vi "Read.vi"(5 "CS Channel":u8, 7 "SPI Channel (0)":u8, 8 "Error In":errorcluster, 10 "LEDs":enum16{"None", "LD1", "LD2", "Both"}(ring)=enum."LD2", 11 "LINX Resource":T1) -> (0 "Error Out":errorcluster, 1 "Y - Axis":string, 2 "X - Axis":string, 3 "LINX Resource":T1, 4 "Buttons":u8)   [LabVIEW 2020, in "LMH-LINX.lvlib" / "PmodJSTK.lvlib"]
doc: "Sets the state of the LEDs on the PmodJSTK and reads X and Y axis data and button values."
uses:
  PmodJSTK.lvlib
  Private/Type Defs/LINX Ref.ctl
  Private/Type Defs/Platform.ctl
  Private/Type Defs/Interface.ctl
  Private/Device/Type Defs/LINX Device Config.ctl
  Private/Device/Type Defs/TCP Config.ctl
  Private/Device/Type Defs/Channels.ctl
  Peripherals/SPI/SPI CS Config.ctl
  Private/Type Defs/Peripherals/SPI/SPI CS Logic Level.ctl
  Peripherals/SPI/SPI Write Read 1 Frame.vi
  Peripherals/SPI/SPI Write Read N Frames.vi
  Utilities/Check Channel.vi
  Private/Utilties/Generate Error.vi
  LMH-LINX.lvlib
  Private/Device/Device.lvlib
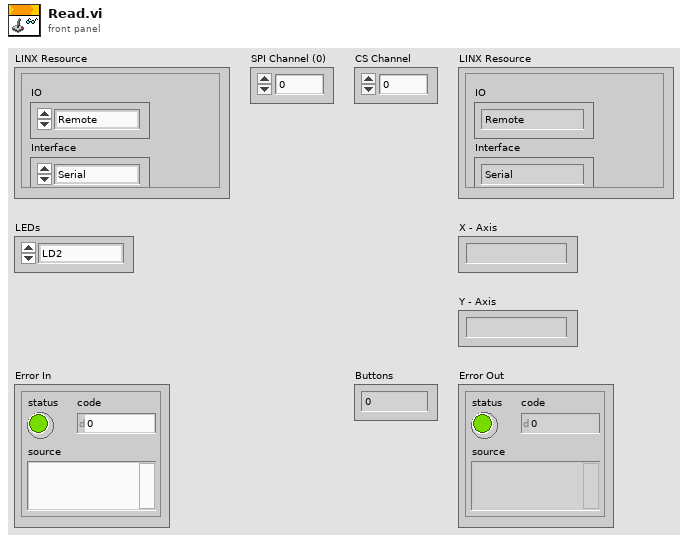
[diagram p1: front panel]
types:
  T1 = typedef "LMH-LINX.lvlib/LINX Ref.ctl" = cluster{"IO":T2, "Interface":T3, "LINX Device Config":T4}
  T2 = typedef "LMH-LINX.lvlib/Platform.ctl" = enum16{"Remote", "Local"}
  T3 = typedef "LMH-LINX.lvlib/Interface.ctl" = enum16{"Serial", "TCP"}
  T4 = typedef "Device.lvlib/LINX Device Config.ctl" = cluster{"Interface":T3, "COM Port":refnum<visa-resource-name>, "TCP Configuration":T5, "Device Family":u8, "Device ID":u8, "Device Name":string, "TCP Ref":refnum<k5>, "Channels":T6}
  T5 = typedef "Device.lvlib/TCP Config.ctl" = cluster{"IP Address":string, "Port":u16}
  T6 = typedef "LMH-LINX.lvlib/Channels.ctl" = cluster{"DI":u8[], "DO":u8[], "AI":u8[], "AO":u8[], "PWM":u8[], "QE":u8[], "UART":u8[], "I2C 2":u8[], "SPI":u8[], "CAN":u8[], "Servo":u8[], "AI Ref (V)":dbl, "AI Resolution (Bits)":u8, "AO Ref (V)":dbl, "AO Resolution (Bits)":u8}
  T7 = typedef "LMH-LINX.lvlib/SPI CS Config.ctl" = cluster{"CS Channel":u8, "CS Logic Level":T8}
  T8 = typedef "LMH-LINX.lvlib/SPI CS Logic Level.ctl" = enum8{"Active Low", "Active High"}
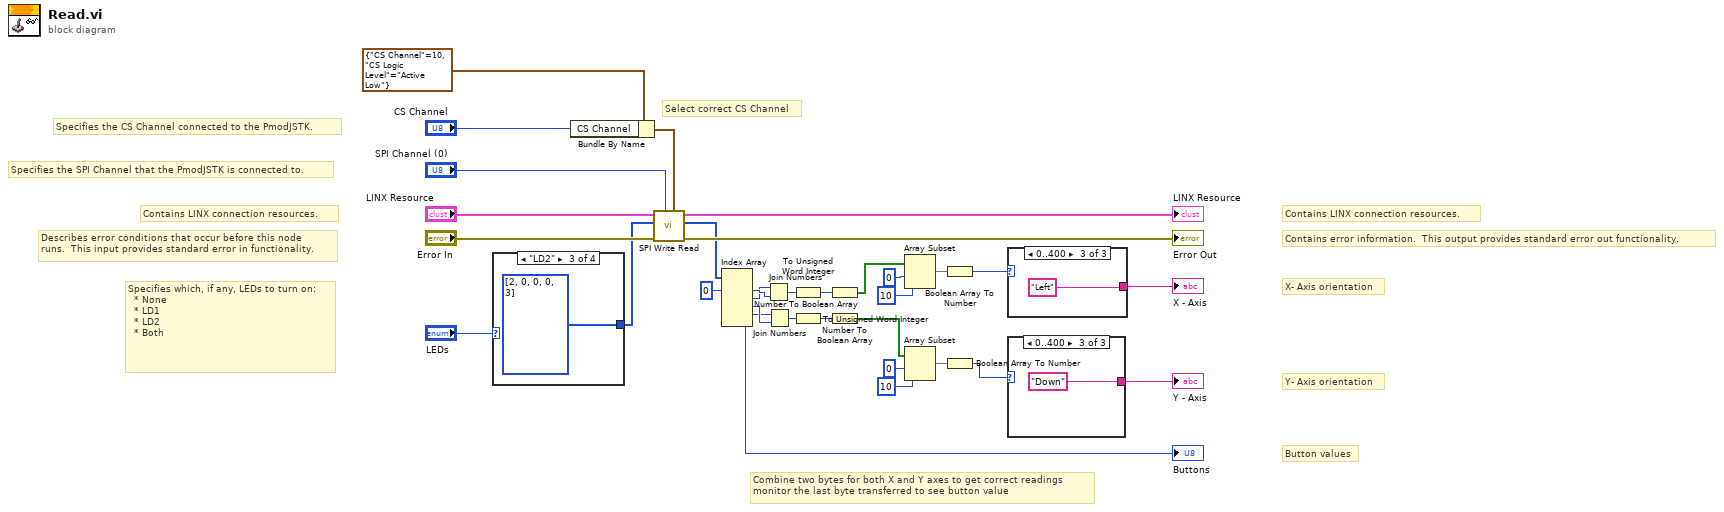
[diagram p0: block diagram]
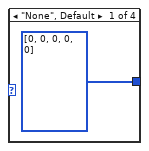
[diagram p2: hidden frame]
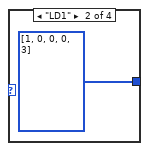
[diagram p3: hidden frame]
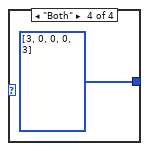
[diagram p4: hidden frame]
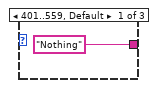
[diagram p5: hidden frame]
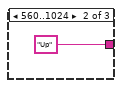
[diagram p6: hidden frame]
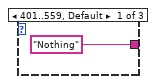
[diagram p7: hidden frame]
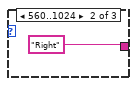
[diagram p8: hidden frame]
diagram:
  # "Specifies which, if any, LEDs to turn on:\n  * None\n  * LD1\n  * LD2\n  * Both"
  # "Specifies the CS Channel connected to the PmodJSTK."
  # "Button values"
  # "Y- Axis orientation"
  # "X- Axis orientation"
  # "Contains error information.  This output provides standard error out functionality."
  # "Contains LINX connection resources."
  # "Describes error conditions that occur before this node\nruns.  This input provides standard error in functionality."
  # "Contains LINX connection resources."
  # "Specifies the SPI Channel that the PmodJSTK is connected to."
  # "Combine two bytes for both X and Y axes to get correct readings\nmonitor the last byte transferred to see button value"
  # "Select correct CS Channel"
  n1 = case shown="\"LD2\"" "LEDs" {
    tunnel: [u8[] [0, 0, 0, 0, 0] u8[] [1, 0, 0, 0, 3] u8[] [2, 0, 0, 0, 3] u8[] [3, 0, 0, 0, 3]] -> w1
    frame "None", Default {
    }
    frame "LD1" {
    }
    frame "LD2" {
    }
    frame "Both" {
    }
  }
  n2 = Bundle By Name(cluster=T7 {"CS Channel"=10, "CS Logic Level"=enum."Active Low"} ("CS Configuration"), "CS Channel"="CS Channel") -> (w33:T7)
  n3 = call-poly "SPI Write Read.vi"("CS Configuration"=w33, "SPI Channel (0)"="SPI Channel (0)", "Error In"="Error In", "Data"=w1, "LINX Resource"="LINX Resource") -> ("Error Out"=→"Error Out":errorcluster, "Read Data"=w9:u8[], "LINX Resource"=→"LINX Resource":T1)  [unwired: 3 in, 1 out]
  n4 = Index Array(array=w9, index #1=0 ("index")) -> (element #1=w12:u8, element #2=w11:u8, element #3=w14:u8, element #4=w13:u8, element #5=→"Buttons":u8)  [unwired: 4 in]
  n5 = Join Numbers(hi=w11, lo=w12) -> ((hi.lo)=w15:u16)
  n6 = Join Numbers(hi=w13, lo=w14) -> ((hi.lo)=w16:u16)
  n7 = To Unsigned Word Integer(number=w15) -> (unsigned 16bit integer=w18:u16)
  n8 = To Unsigned Word Integer(number=w16) -> (unsigned 16bit integer=w17:u16)
  n9 = Number To Boolean Array(number=w18) -> (Boolean array=w19:bool[])
  n10 = Number To Boolean Array(number=w17) -> (Boolean array=w20:bool[])
  n11 = Array Subset(array=w19, index=0, length=10) -> (w25:bool[])
  n12 = Array Subset(array=w20, index=0, length=10) -> (w29:bool[])
  n13 = Boolean Array To Number(Boolean array=w25) -> (number=w26:u32)
  n14 = Boolean Array To Number(Boolean array=w29) -> (number=w27:u32)
  n15 = case shown="0..400" w26 {
    tunnel: ["Nothing" "Right" "Left"] -> w30
    frame 401..559, Default {
    }
    frame 560..1024 {
    }
    frame 0..400 {
    }
  }
  "X - Axis" <- w30
  n16 = case shown="0..400" w27 {
    tunnel: ["Nothing" "Up" "Down"] -> w31
    frame 401..559, Default {
    }
    frame 560..1024 {
    }
    frame 0..400 {
    }
  }
  "Y - Axis" <- w31
